vi "Data Sensor.vi"(0 "VISA resource name":refnum<visa-resource-name>, 7 "Input (0: A)":u16(ring) items=["A", "B", "C", "D"], 11 "error in (no error)":errorcluster) -> (4 "VISA resource name out":refnum<visa-resource-name>, 6 "Celsius Reading":dbl min=-273.16 max=1372.0 step=1e-05 format="%^.5e", 8 "Kelvin Reading":dbl min=0.0 max=1645.0 step=1e-05 format="%^.5e", 10 "Sensor Units Reading":dbl min=-7.5 max=300000.0 step=1e-05 format="%^.5e", 15 "error out":errorcluster)   [LabVIEW 2019, in "Lake Shore Cryotronics 340.lvlib"]
doc: "This VI querys the instrument for an inputs sensor reading in Celsius, Kelvin, and Sensor Units."
uses:
  Lake Shore Cryotronics 340.lvlib
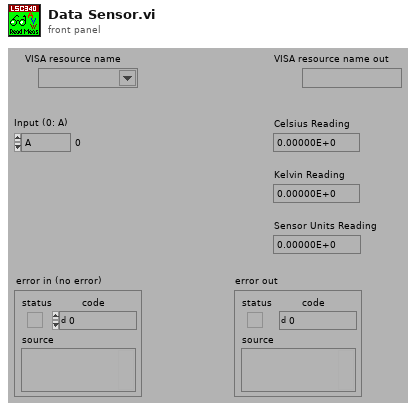
[diagram p1: front panel]
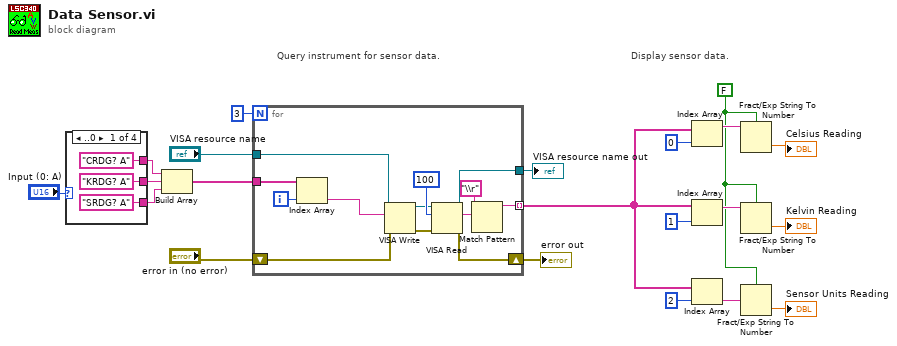
[diagram p0: block diagram]
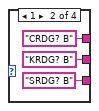
[diagram p2: hidden frame]
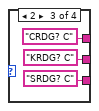
[diagram p3: hidden frame]
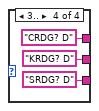
[diagram p4: hidden frame]
diagram:
  w1 = FALSE ("use system decimal point (T)")
  # "Query instrument for sensor data."
  # "Display sensor data."
  n1 = case shown="..0" "Input (0: A)" {
    tunnel: ["CRDG? A" "CRDG? B" "CRDG? C" "CRDG? D"] -> w10
    tunnel: ["KRDG? A" "KRDG? B" "KRDG? C" "KRDG? D"] -> w9
    tunnel: ["SRDG? A" "SRDG? B" "SRDG? C" "SRDG? D"] -> w8
    frame ..0 {
    }
    frame 1 {
    }
    frame 2 {
    }
    frame 3.. {
    }
  }
  n2 = Build Array(w10, w9, w8) -> (w11:string[])
  n3 = for {
    N: 3 -> [_]
    tunnel: w11 -> [w43]
    shift-right: [w40] -> w4
    shift-left: "error in (no error)" -> [w41]
    tunnel: [w39] -> w3
    tunnel: "VISA resource name" -> [w38]
    tunnel: [w36] -> w2 mode=indexing
    i -> [w42]
    n4 = Index Array(array=w43, index=w42) -> (element=w34:string)
    n5 = VISA Write(VISA resource name=w38, write buffer=w34, error in (no error)=w41) -> (VISA resource name out=w35:refnum<visa-resource-name>, error out=w46:errorcluster)  [unwired: 1 out]
    n6 = VISA Read(VISA resource name=w35, byte count=100, error in (no error)=w46) -> (VISA resource name out=w39:refnum<visa-resource-name>, read buffer=w44:string, error out=w40:errorcluster)  [unwired: 1 out]
    n7 = Match Pattern(string=w44, regular expression="\\r") -> (before substring=w36:string)  [unwired: 1 in, 3 out]
  }
  "VISA resource name out" <- w3
  "error out" <- w4
  n8 = Index Array(array=w2, index=0) -> (element=w16:string)
  n9 = Index Array(array=w2, index=1) -> (element=w17:string)
  n10 = Index Array(array=w2, index=2) -> (element=w18:string)
  n11 = Fract/Exp String To Number(use system decimal point (T)=w1, string=w16) -> (number=→"Celsius Reading":dbl)  [unwired: 2 in, 1 out]
  n12 = Fract/Exp String To Number(use system decimal point (T)=w1, string=w17) -> (number=→"Kelvin Reading":dbl)  [unwired: 2 in, 1 out]
  n13 = Fract/Exp String To Number(use system decimal point (T)=w1, string=w18) -> (number=→"Sensor Units Reading":dbl)  [unwired: 2 in, 1 out]
